vi "Sequence Retrieve Record.vi"(8 "error in (no error)":errorcluster, 11 "Statement Refnum":T1) -> (0 "error out":errorcluster, 2 "Sequence Record":T2, 3 "Statement Refnum":T1)   [LabVIEW 2011]
uses:
  Sequence Record.ctl
  Summitek EXT/ODBC/SQL Controls/Statement Refnum.ctl
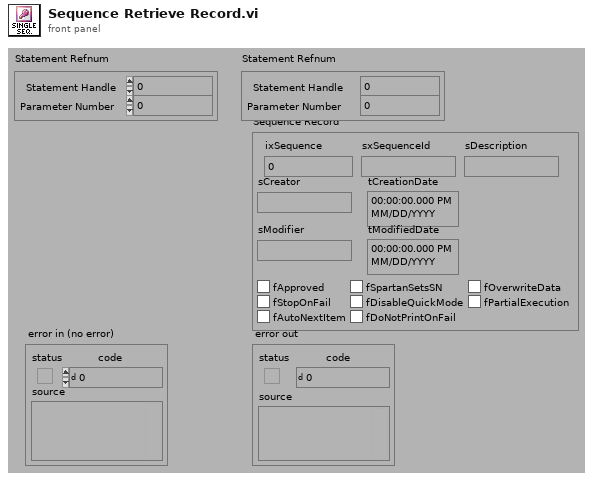
[diagram p1: front panel]
types:
  T1 = typedef "Statement Refnum.ctl" = cluster{"Statement Handle":i32, "Parameter Number":u16}
  T2 = typedef "Sequence Record.ctl" = cluster{"ixSequence":i32, "sxSequenceId":string, "sDescription":string, "sCreator":string, "tCreationDate":timestamp, "sModifier":string, "tModifiedDate":timestamp, "fApproved":bool, "fSpartanSetsSN":bool, "fOverwriteData":bool, "fStopOnFail":bool, "fDisableQuickMode":bool, "fPartialExecution":bool, "fAutoNextItem":bool, "fDoNotPrintOnFail":bool}
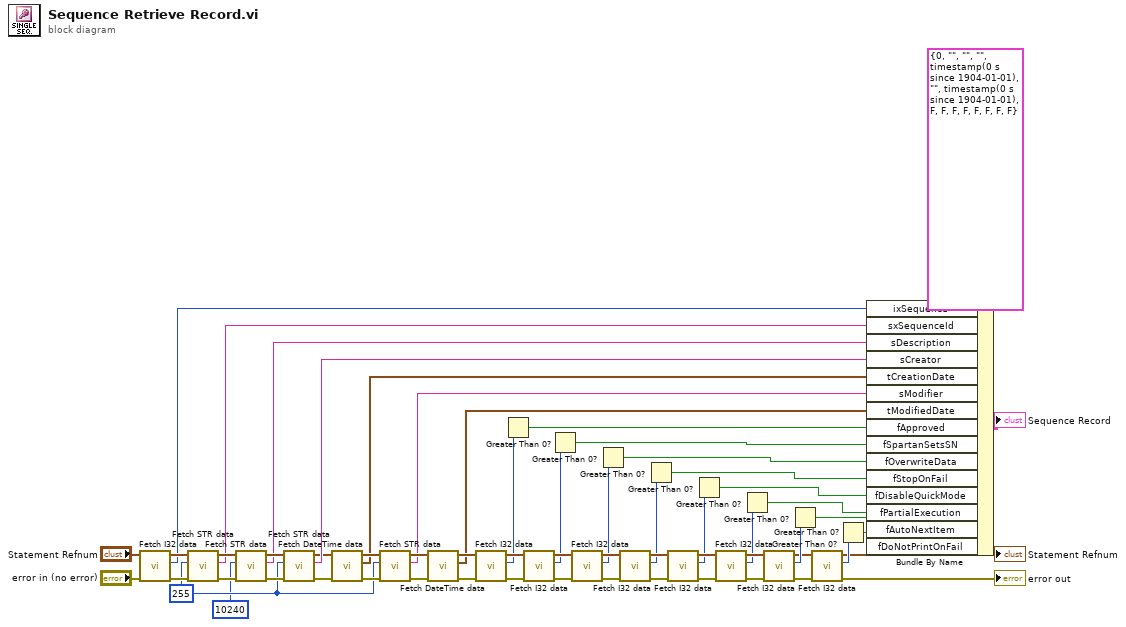
[diagram p0: block diagram]
diagram:
  w27 = 255 ("Buffer Size")
  n1 = call "Fetch I32 data.vi"("error in (no error)"="error in (no error)", "Statement Refnum"="Statement Refnum") -> ("error out"=w47:errorcluster, "Data"=w46:i32, "Statement Refnum"=w48:T1)  [unwired: 3 out]
  n2 = call "Fetch STR data.vi"("error in (no error)"=w47, "Buffer Size"=w27, "Statement Refnum"=w48) -> ("error out"=w59:errorcluster, "Data"=w55:string, "Statement Refnum"=w58:T1)  [unwired: 2 out]
  n3 = call "Fetch STR data.vi"("error in (no error)"=w59, "Buffer Size"=10240, "Statement Refnum"=w58) -> ("error out"=w57:errorcluster, "Data"=w54:string, "Statement Refnum"=w56:T1)  [unwired: 2 out]
  n4 = call "Fetch STR data.vi"("error in (no error)"=w57, "Buffer Size"=w27, "Statement Refnum"=w56) -> ("error out"=w44:errorcluster, "Data"=w53:string, "Statement Refnum"=w45:T1)  [unwired: 2 out]
  n5 = call "Fetch DateTime data.vi"("error in (no error)"=w44, "Statement Refnum"=w45) -> ("error out"=w28:errorcluster, "Data"=w11:timestamp, "Statement Refnum"=w39:T1)  [unwired: 3 out]
  n6 = call "Fetch STR data.vi"("error in (no error)"=w28, "Buffer Size"=w27, "Statement Refnum"=w39) -> ("error out"=w29:errorcluster, "Data"=w26:string, "Statement Refnum"=w38:T1)  [unwired: 2 out]
  n7 = call "Fetch DateTime data.vi"("error in (no error)"=w29, "Statement Refnum"=w38) -> ("error out"=w30:errorcluster, "Data"=w10:timestamp, "Statement Refnum"=w37:T1)  [unwired: 3 out]
  n8 = call "Fetch I32 data.vi"("error in (no error)"=w30, "Statement Refnum"=w37) -> ("error out"=w52:errorcluster, "Data"=w25:i32, "Statement Refnum"=w51:T1)  [unwired: 3 out]
  n9 = Greater Than 0?(x=w25) -> (x > 0?=w24:bool)
  n10 = call "Fetch I32 data.vi"("error in (no error)"=w52, "Statement Refnum"=w51) -> ("error out"=w31:errorcluster, "Data"=w18:i32, "Statement Refnum"=w36:T1)  [unwired: 3 out]
  n11 = Greater Than 0?(x=w18) -> (x > 0?=w12:bool)
  n12 = call "Fetch I32 data.vi"("error in (no error)"=w31, "Statement Refnum"=w36) -> ("error out"=w42:errorcluster, "Data"=w19:i32, "Statement Refnum"=w43:T1)  [unwired: 3 out]
  n13 = Greater Than 0?(x=w19) -> (x > 0?=w13:bool)
  n14 = call "Fetch I32 data.vi"("error in (no error)"=w42, "Statement Refnum"=w43) -> ("error out"=w32:errorcluster, "Data"=w20:i32, "Statement Refnum"=w35:T1)  [unwired: 3 out]
  n15 = Greater Than 0?(x=w20) -> (x > 0?=w14:bool)
  n16 = call "Fetch I32 data.vi"("error in (no error)"=w32, "Statement Refnum"=w35) -> ("error out"=w41:errorcluster, "Data"=w21:i32, "Statement Refnum"=w40:T1)  [unwired: 3 out]
  n17 = Greater Than 0?(x=w21) -> (x > 0?=w15:bool)
  n18 = call "Fetch I32 data.vi"("error in (no error)"=w41, "Statement Refnum"=w40) -> ("error out"=w33:errorcluster, "Data"=w22:i32, "Statement Refnum"=w34:T1)  [unwired: 3 out]
  n19 = Greater Than 0?(x=w22) -> (x > 0?=w16:bool)
  n20 = call "Fetch I32 data.vi"("error in (no error)"=w33, "Statement Refnum"=w34) -> ("error out"=w4:errorcluster, "Data"=w23:i32, "Statement Refnum"=w5:T1)  [unwired: 3 out]
  n21 = Greater Than 0?(x=w23) -> (x > 0?=w17:bool)
  n22 = call "Fetch I32 data.vi"("error in (no error)"=w4, "Statement Refnum"=w5) -> ("error out"=→"error out":errorcluster, "Data"=w6:i32, "Statement Refnum"=→"Statement Refnum":T1)  [unwired: 3 out]
  n23 = Greater Than 0?(x=w6) -> (x > 0?=w1:bool)
  n24 = Bundle By Name(cluster=T2 {"ixSequence"=0, "sxSequenceId"="", "sDescription"="", "sCreator"="", "tCreationDate"=timestamp(0 s since 1904-01-01), "sModifier"="", "tModifiedDate"=timestamp(0 s since 1904-01-01), "fApproved"=FALSE, "fSpartanSetsSN"=FALSE, "fOverwriteData"=FALSE, "fStopOnFail"=FALSE, "fDisableQuickMode"=FALSE, "fPartialExecution"=FALSE, "fAutoNextItem"=FALSE, "fDoNotPrintOnFail"=FALSE} ("Sequence Data"), "ixSequence"=w46, "sxSequenceId"=w55, "sDescription"=w54, "sCreator"=w53, "tCreationDate"=w11, "sModifier"=w26, "tModifiedDate"=w10, "fApproved"=w24, "fSpartanSetsSN"=w12, "fOverwriteData"=w13, "fStopOnFail"=w14, "fDisableQuickMode"=w15, "fPartialExecution"=w16, "fAutoNextItem"=w17, "fDoNotPrintOnFail"=w1) -> (→"Sequence Record":T2)
